vi "簇捆绑松绑.vi"() -> ()   [LabVIEW 2020]
doc: "本VI是为《我和LabVIEW》一书编写的示例。\n关于本书的介绍请参考网页：\nhttp://ruanqizhen.spaces.live.com/blog/cns!5852D4F797C53FB6!4310.entry"
panel:
  in  "error in (no error) 2":errorcluster caption="错误输入（无错误）"
  out "error out 2":errorcluster caption="错误输出"
  out "error out":errorcluster caption="错误输出"
  in  "error in (no error)":errorcluster caption="错误输入（无错误）"
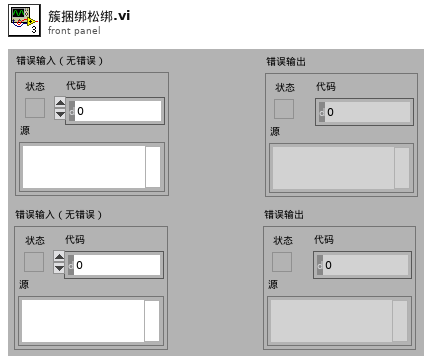
[diagram p1: front panel]
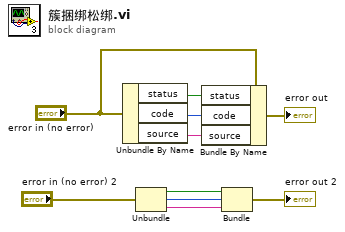
[diagram p0: block diagram]
diagram:
  n1 = Unbundle By Name("error in (no error)") -> ("status"=w9:bool, "code"=w8:i32, "source"=w7:string)
  n2 = Unbundle("error in (no error) 2") -> ("status"=w5:bool, "code"=w4:i32, "source"=w3:string)
  n3 = Bundle By Name(cluster="error in (no error)", "status"=w9, "code"=w8, "source"=w7) -> (→"error out":errorcluster)
  n4 = Bundle("status"=w5, "code"=w4, "source"=w3) -> (→"error out 2":errorcluster)  [unwired: 1 in]
